vi "Apply Theme To TitleBar-Pane.vi"(8 "Error In":errorcluster, 9 "Override Root With (Empty)":string, 10 "TitleBar Pane Refs":refnum<vi>[](array[refnum]), 11 "ini Theme in":refnum<class "ini Theme.lvclass">) -> (0 "Error Out":errorcluster, 3 "ini Theme out":refnum<class "ini Theme.lvclass">)   [LabVIEW 2021, in "Appearance Actor.lvlib" / "ini Theme.lvclass"]
uses:
  ini Theme.lvclass
  Generic Theme/API/Typedefs/Theme Entry--enum.ctl
  ini Theme.lvclass/ini Theme.ctl
  fa3b262b-9dee-4a2a-a40e-e8b24c2842d1.vi
  e580e7d3-37e0-4797-b7d4-6ea3cff1905c.vi
  <vilib>/Utility/config.llb/Read Key (U32).vi
  <vilib>/Utility/config.llb/NI_LVConfig.lvlib
  Generic Theme/Generic Theme.lvclass
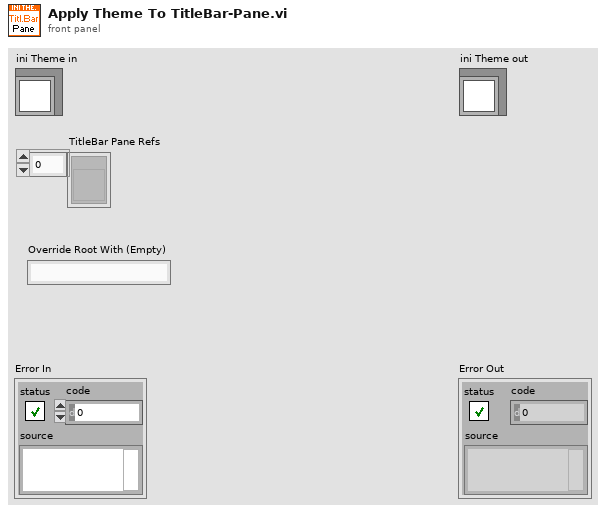
[diagram p1: front panel]
types:
  T1 = typedef "Appearance Actor.lvlib/Generic Theme.lvclass/Theme Entry--enum.ctl" = enum16{"None", "TitleBar.Pane.Color", "TitleBar.Splitter.FillColor", "TitleBar.Splitter.OutlineColor", "TitleBar.Title.Font.Color", "TitleBar.Title.Font.Family", "TitleBar.Title.Font.Size", "TitleBar.Title.Font.Style"}
  T2 = typedef "NI_LVConfig.lvlib/Config Data RefNum.ctl" = refnum<k1>
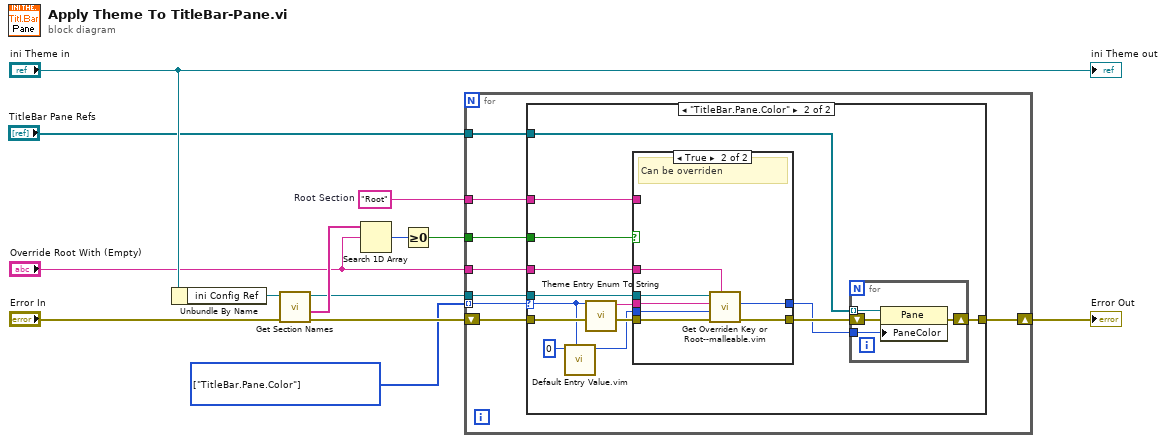
[diagram p0: block diagram]
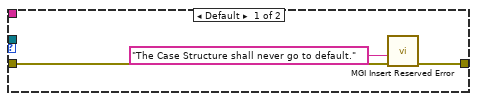
[diagram p2: hidden frame]
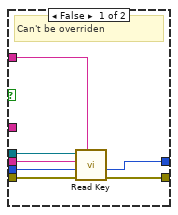
[diagram p3: hidden frame]
diagram:
  w2 = T1[] [enum."TitleBar.Pane.Color"] items=["None", "TitleBar.Pane.Color", "TitleBar.Splitter.FillColor", "TitleBar.Splitter.OutlineColor", "TitleBar.Title.Font.Color", "TitleBar.Title.Font.Family", "TitleBar.Title.Font.Size", "TitleBar.Title.Font.Style"] ("Array")
  w3 = "Root"  # Root Section
  n1 = Unbundle By Name("ini Theme in") -> ("ini Config Ref"=w13:T2)
  n2 = call <vilib>:"Get Section Names.vi"("error in (no error)"="Error In", "refnum"=w13) -> ("error out"=w10:errorcluster, "section names"=w12:string[], "refnum out"=w4:T2)  [unwired: 7 in]
  n3 = Search 1D Array(1D array=w12, element="Override Root With (Empty)") -> (index of element=w11:i32)  [unwired: 1 in]
  n4 = Greater Or Equal To 0?(x=w11) -> (x >= 0?=w5:bool)
  n5 = for {
    shift-right: [w15] -> w8
    shift-left: w10 -> [w21]
    tunnel: "Override Root With (Empty)" -> [w20]
    tunnel: w5 -> [w19]
    tunnel: w4 -> [w18]
    tunnel: w3 -> [w17]
    tunnel: w2 -> [w16] mode=indexing
    tunnel: "TitleBar Pane Refs" -> [w14]
    n6 = case shown="\"TitleBar.Pane.Color\"" w16 {
      selector: w16 -> [_ w27]
      tunnel: w21 -> [w23 w37]
      tunnel: w20 -> [_ w35]
      tunnel: w19 -> [_ w34]
      tunnel: w18 -> [_ w33]
      tunnel: w17 -> [_ w32]
      tunnel: [w22 w31] -> w15
      tunnel: w14 -> [_ w30]
      frame Default {
        n7 = call <userlib>:"MGI Insert Reserved Error.vi"("Error In"=w23, "Error Description"="The Case Structure shall never go to default.") -> ("Error Out"=w22:errorcluster)  [unwired: 9 in]
      }
      frame "TitleBar.Pane.Color" {
        n8 = call "Default Entry Value.vim"("Root Theme Entry"=w27, "Data Type"=u32 0) -> ("Default Value"=w26:u32)  [unwired: 9 in]
        n9 = call "Theme Entry Enum To String.vi"("Root Theme Entry"=w27) -> ("Root Theme Entry String"=w28:string)  [unwired: 10 in]
        n10 = case shown="True" w34 {
          tunnel: w37 -> [w48 w55]
          tunnel: [w47 w54] -> w36
          tunnel: w35 -> [_ w53]
          tunnel: w33 -> [w45 w52]
          tunnel: w32 -> [w46 _]
          tunnel: w28 -> [w44 w51]
          tunnel: w26 -> [w42 w50]
          tunnel: [w43 w49] -> w29
          frame False {
            # "Can't be overriden"
            n11 = call-poly <vilib>:"Read Key.vi"("section"=w46, "error in (no error)"=w48, "default value"=w42, "key"=w44, "refnum"=w45) -> ("error out"=w47:errorcluster, "value"=w43:u32)  [unwired: 3 in, 2 out]
          }
          frame True {
            # "Can be overriden"
            n12 = call "Get Overriden Key or Root--malleable.vim"("Override Root With"=w53, "Error In"=w55, "Default"=w50, "Key"=w51, "ini Ref In"=w52) -> ("Error Out"=w54:errorcluster, "Value"=w49:u32)  [unwired: 4 in, 1 out]
          }
        }
        n13 = for {
          tunnel: w30 -> [w39] mode=indexing
          tunnel: w29 -> [w38]
          shift-right: [w40] -> w31
          shift-left: w36 -> [w41]
          n14 = property class="Pane"(reference=w39, error in=w41, "PaneColor"=w38) -> (error out=w40:errorcluster)  [unwired: 1 out]
        }
      }
    }
  }
  "Error Out" <- w8
  "ini Theme out" <- "ini Theme in"
